vi "BlueMiddleAutos.vi"() -> (3 "Auto Ran":string)   [LabVIEW 2016]
uses:
  <vilib>/Rock Robotics/Network Tables/NT Read String.vi
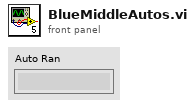
[diagram p1: front panel]
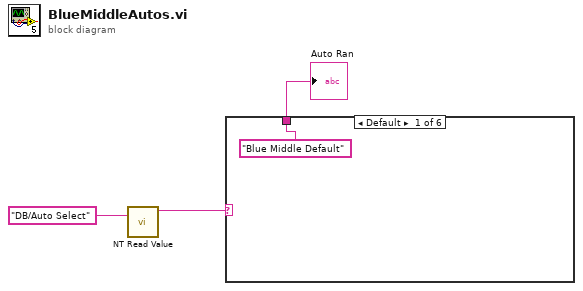
[diagram p0: block diagram]
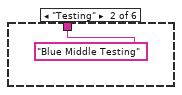
[diagram p2: hidden frame]
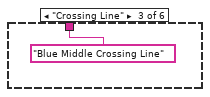
[diagram p3: hidden frame]
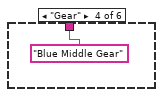
[diagram p4: hidden frame]
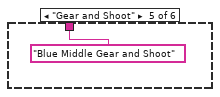
[diagram p5: hidden frame]
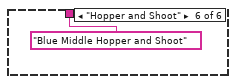
[diagram p6: hidden frame]
diagram:
  n1 = call-poly <vilib>:"NT Read Value.vi"("Name"="DB/Auto Select") -> ("String"=w2:string)  [unwired: 9 in, 1 out]
  n2 = case shown="Default" w2 {
    tunnel: ["Blue Middle Default" "Blue Middle Testing" "Blue Middle Crossing Line" "Blue Middle Gear" "Blue Middle Gear and Shoot" "Blue Middle Hopper and Shoot"] -> w1
    frame Default {
    }
    frame "Testing" {
    }
    frame "Crossing Line" {
    }
    frame "Gear" {
    }
    frame "Gear and Shoot" {
    }
    frame "Hopper and Shoot" {
    }
  }
  "Auto Ran" <- w1
